vi "Arrange Array.vi"(1 "Order":string[](array[string]), 2 "Arrange array":T1(array[cluster])) -> (0 "Arranged array":T1(array[cluster]))   [LabVIEW 2013]
doc: "This VI arranges an array in a specific order based on each element's name."
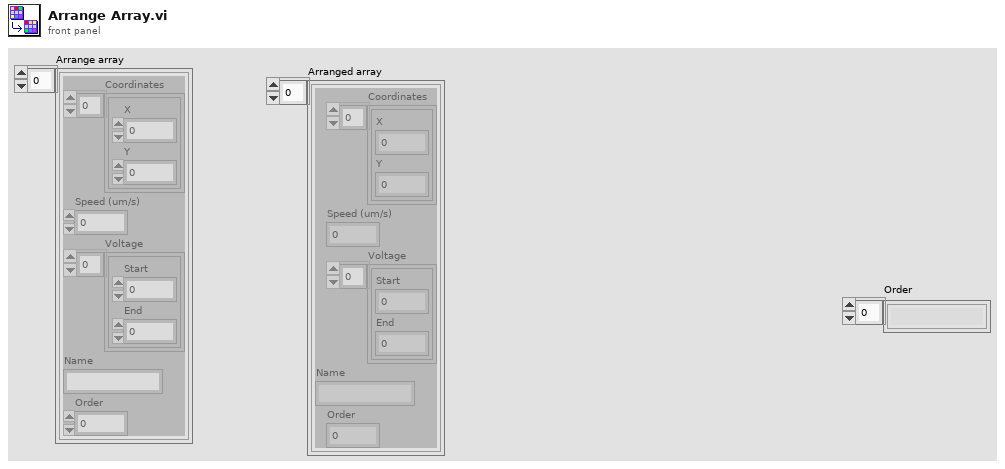
[diagram p1: front panel]
types:
  T1 = cluster{"Coordinates":cluster{"X":dbl, "Y":dbl}[], "Speed (um/s)":dbl, "Voltage":cluster{"Start":dbl, "End":dbl}[], "Name":string, "Order":i32}[]
  T2 = cluster{"Coordinates":cluster{"X":dbl, "Y":dbl}[], "Speed (um/s)":dbl, "Voltage":cluster{"Start":dbl, "End":dbl}[], "Name":string, "Order":i32}
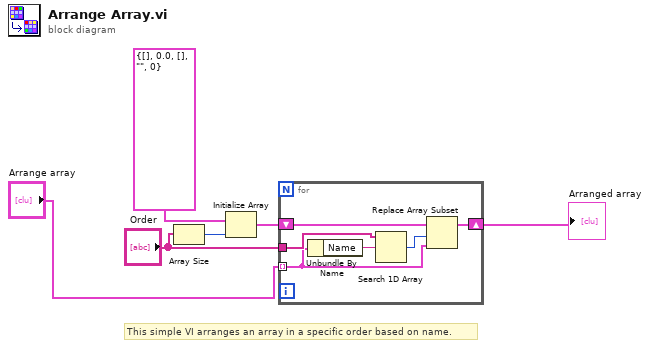
[diagram p0: block diagram]
diagram:
  # "This simple VI arranges an array in a specific order based on name."
  n1 = Array Size(array="Order") -> (size(s)=w6:i32)
  n2 = Initialize Array(T2 {"Coordinates"=[], "Speed (um/s)"=0.0, "Voltage"=[], "Name"="", "Order"=0}, w6) -> (w4:T1)
  n3 = for {
    tunnel: "Arrange array" -> [w9] mode=indexing
    tunnel: "Order" -> [w11]
    shift-right: [w8] -> w2
    shift-left: w4 -> [w7]
    n4 = Unbundle By Name(w9) -> ("Name"=w10:string)
    n5 = Search 1D Array(1D array=w11, element=w10) -> (index of element=w12:i32)  [unwired: 1 in]
    n6 = Replace Array Subset(array=w7, new element=w9, index=w12) -> (w8:T1)
  }
  "Arranged array" <- w2
